vi "GetText.vi"(8 "error in":errorcluster, 11 "node in":refnum<class "Device.lvclass">) -> (0 "error out":errorcluster, 1 "additional text":string, 2 "text":string, 3 "node out":refnum<class "Device.lvclass">, 4 "glyph":string)   [LabVIEW 2014, in "Device.lvclass"]
doc: "Returns the text representation of the node used for the tree control."
uses:
  Device.lvclass
  Device.lvclass/Device.ctl
  <vilib>/NI/Configuration Framework/serializable configuration/NISE_CEF_serializable configuration.lvclass
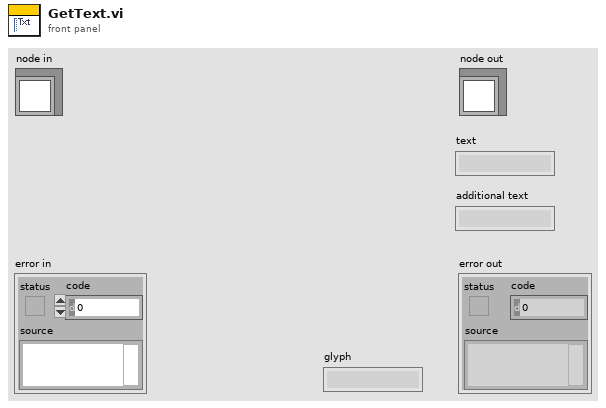
[diagram p1: front panel]
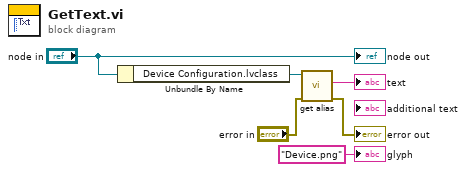
[diagram p0: block diagram]
diagram:
  n1 = Unbundle By Name("node in") -> ("Device Configuration.lvclass"=w4:refnum<class "Device Configuration.lvclass">)
  n2 = call <vilib>:"get alias.vi"("error in"="error in", "configuration in"=w4) -> ("error out"=→"error out":errorcluster, "alias"=→"text":string)  [unwired: 7 in, 1 out]
  "node out" <- "node in"
  "glyph" <- "Device.png" ("glyph")
